vi "NewGame.vi"(7 "TetrisType (ChildObject)":refnum<class "Tetris.lvclass">, 8 "error in (no error)":errorcluster, 11 "FPGA_ref":T1) -> (0 "error out":errorcluster, 3 "Tetris out":refnum<class "Tetris.lvclass">)   [LabVIEW 2019, in "RT_Game.lvlib" / "Tetris.lvclass"]
uses:
  Tetris.lvclass
  FPGA_Interface.ctl
  Game/Game.lvclass
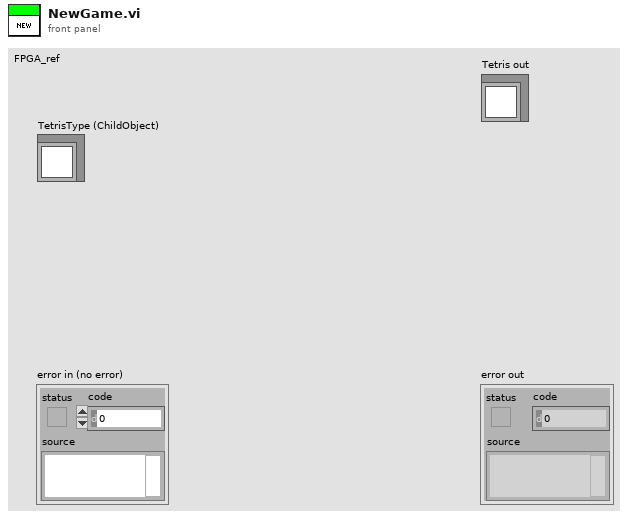
[diagram p1: front panel]
types:
  T1 = typedef "FPGA_Interface.ctl" = refnum<k20>
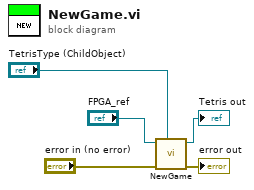
[diagram p0: block diagram]
diagram:
  n1 = call-parent "NewGame.vi"("GameType (ChildObject)"="TetrisType (ChildObject)", "error in (no error)"="error in (no error)", "FPGA_ref"="FPGA_ref") -> ("error out"=→"error out":errorcluster, "Game out"=→"Tetris out":refnum<class "Tetris.lvclass">)  [unwired: 7 in]
